vi "Task 2 bling.vi"() -> ()   [LabVIEW 2021]
panel:
  in  "?":bool
  in  "stop":bool
  out "led 1":bool
  out "led 2":bool
  out "led 4":bool
  out "led 8":bool
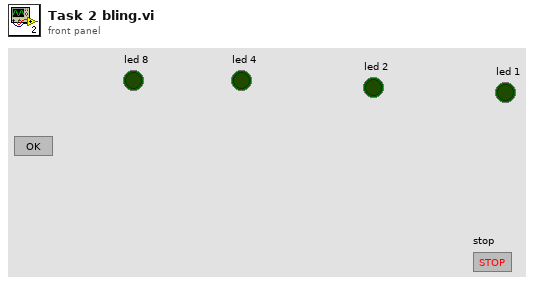
[diagram p1: front panel]
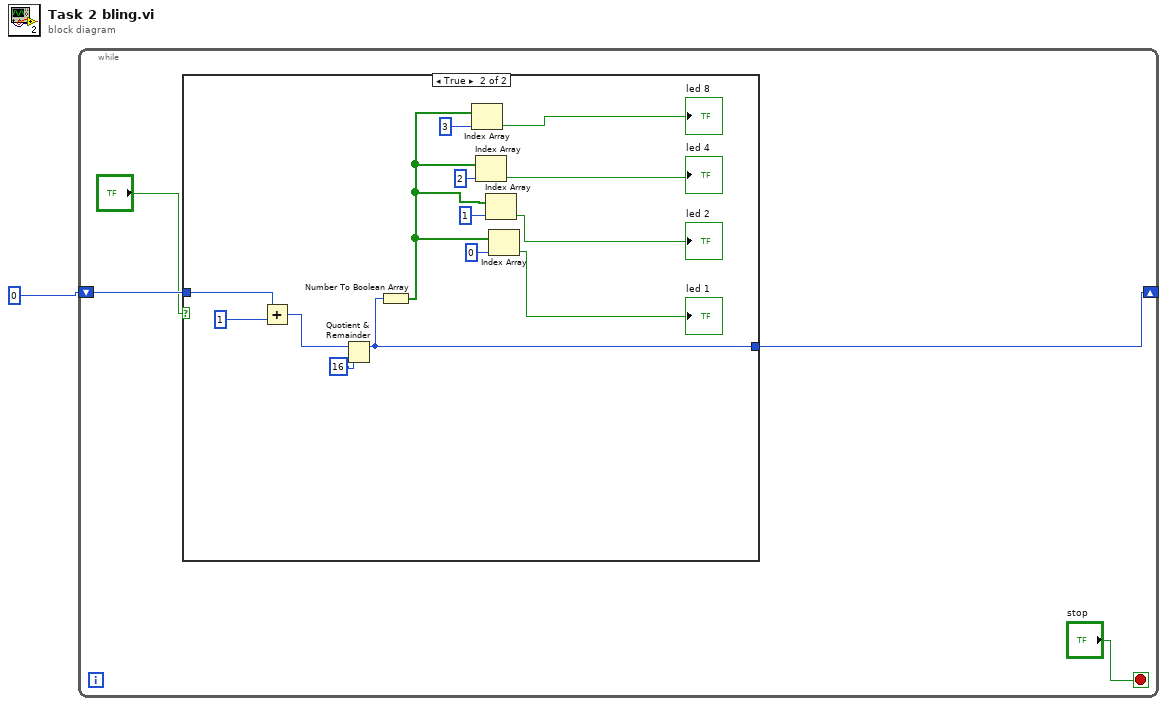
[diagram p0: block diagram]
diagram:
  n1 = while {
    shift-right: [w4] -> _
    shift-left: 0 -> [w5]
    stop <- "stop" stop-if-true
    n2 = case shown="True" "?" {
      tunnel: w5 -> [w6 w20]
      tunnel: [w6 w17] -> w4
      frame False {
      }
      frame True {
        n3 = Add(x=w20, y=1) -> (x+y=w18:i32)
        n4 = Quotient & Remainder(x=w18, y=16) -> (x-y*floor(x/y)=w17:i32)  [unwired: 1 out]
        n5 = Number To Boolean Array(number=w17) -> (Boolean array=w11:bool[])
        n6 = Index Array(array=w11, index=3) -> (element=→"led 8":bool)
        n7 = Index Array(array=w11, index=2) -> (element=→"led 4":bool)
        n8 = Index Array(array=w11, index=1) -> (element=→"led 2":bool)
        n9 = Index Array(array=w11, index=0) -> (element=→"led 1":bool)
      }
    }
  }
